vi "Stop Acquisition.vi"(8 "error in (no error)":cluster{"状态":bool, "代码":i32, "源":string} caption="错误输入（无错误）", 11 "硬件资源输入":T1) -> (0 "error out":cluster{"状态":bool, "代码":i32, "源":string} caption="错误输出")   [LabVIEW 2012, in "Acquisition.lvlib"]
doc: "停止采集。"
uses:
  Acquisition.lvlib
  Hardware Configuration.ctl
  Signal Type.ctl
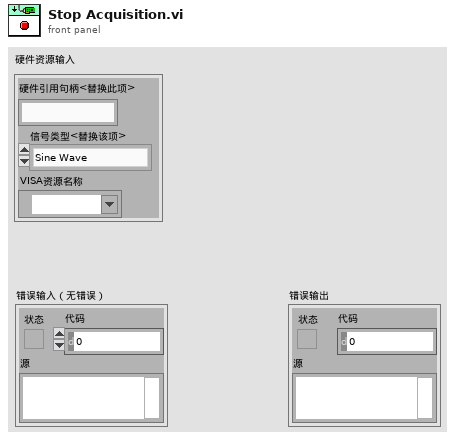
[diagram p1: front panel]
types:
  T1 = typedef "Acquisition.lvlib/Hardware Configuration.ctl" = cluster{"硬件引用句柄<替换此项>":string, "信号类型<替换该项>":T2, "VISA资源名称":refnum<visa-resource-name>}
  T2 = typedef "Acquisition.lvlib/Signal Type.ctl" = enum16{"Sine Wave", "Square with Noise"}
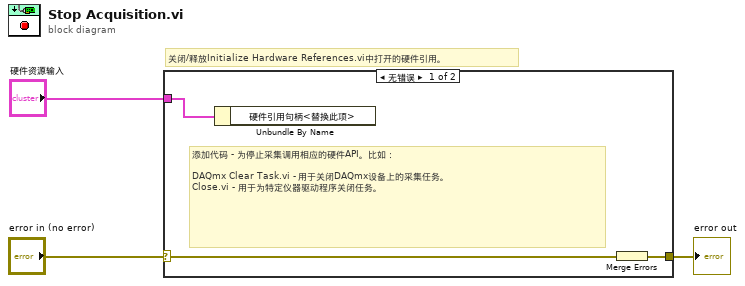
[diagram p0: block diagram]
diagram:
  # "关闭/释放Initialize Hardware References.vi中打开的硬件引用。"
  n1 = case shown="无错误" "error in (no error)" {
    selector: "error in (no error)" -> [w5 w7]
    tunnel: [w6 w7] -> w2
    tunnel: "硬件资源输入" -> [w4 _]
    frame No Error {
      # "添加代码 - 为停止采集调用相应的硬件API。比如：\n\nDAQmx Clear Task.vi - 用于关闭DAQmx设备上的采集任务。\nClose.vi - 用于为特定仪器驱动程序关闭任务。"
      n2 = Unbundle By Name(w4) -> ()  [unwired: 1 out]
      n3 = Merge Errors(w5) -> (w6:errorcluster)
    }
    frame Error {
    }
  }
  "error out" <- w2
